vi "Write Element Selected Event.vi"(4 "error in (no error)":errorcluster, 5 "Value":refnum<user-event>, 6 "Container State":T2, 7 "Display State In":T1) -> (0 "error out":errorcluster, 3 "Display State Out":T1)   [LabVIEW 2015, in "Song Browser.lvlib" / "Song Browser.xctl"]
uses:
  Song Browser.xctl
  <vilib>/_xctls/Container State.ctl
  State.ctl
  controls/Song Browser Display.ctl
  file/MusicElement/Song/Song Duration.ctl
  controls/Enqueue Control.ctl
  <vilib>/_xctls/XControlSupport.lvlib
  file/MusicElement/Song/Song.lvclass
panel:
  # "Replace the Value Control below with a Control of desired type.\nDo not remove this Control or the others from the connector pane.\nDo not change the connector pane pattern.\nThe Value control should always be the third terminal from top on the input side in the connector pane."
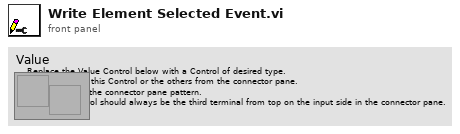
[diagram p1: front panel]
types:
  T1 = typedef "Song Browser.lvlib/Song Browser.xctl/State.ctl" = cluster{"Element Selected Event":refnum<user-event>}
  T2 = typedef "XControlSupport.lvlib/Container State.ctl" = cluster{"Indicator?":bool, "Run Mode?":bool, " Refnum":refnum<vi>}
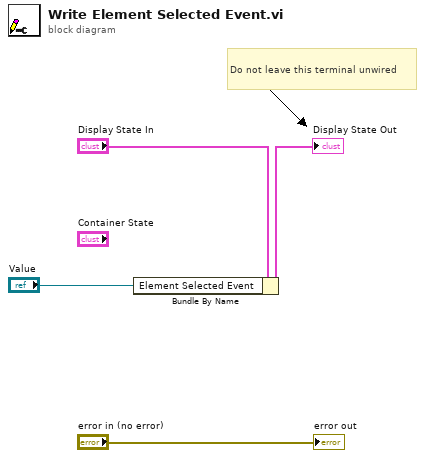
[diagram p0: block diagram]
diagram:
  # "Do not leave this terminal unwired"
  n1 = Bundle By Name(cluster="Display State In", "Element Selected Event"="Value") -> (→"Display State Out":T1)
  "error out" <- "error in (no error)"
